vi "SetCurrentSource.vi"() -> ()   [LabVIEW 2024]
uses:
  <vilib>/Instr/_visa.llb/VISA Configure Serial Port (Instr).vi
  <vilib>/Utility/file.llb/Write Delimited Spreadsheet (DBL).vi
panel:
  out "OPT_PWR_MV":dbl format="%#_13g"
  in  "30 dB Power Conversion Factor":dbl=0.0531
  in  "Signal Scaling Factor":dbl
  in  "20 dB Power Conversion Factor":dbl=0.1692
  out "Settings read string":string
  out "Settings reply":string
  out "Settings string":string
  out "ADC read string":string
  in  "Voltage stop (mV)":dbl=3000.0 format="%#_13g"
  out "Saved location and filename":path
  in  "Filename and location":path
  in  "Cal constant":dbl=1.0 format="%#_13g"
  in  "Loop length (ms)":i32=1000
  in  "Voltage step (mV)":dbl=20.0 format="%#_13g"
  out "Voltage (mV)":dbl
  out "Pulse Width":dbl
  out "Frequency":dbl
  out "ACD 2":dbl
  out "ADC 3":dbl
  out "ADC 4":dbl
  out "ADC 1":dbl
  out "RAW 3":dbl
  out "RAW 2":dbl
  out "RAW 4":dbl
  out "RAW 1":dbl
  out "Running?":bool
  in  "ON/OFF":bool
  in  "Voltage start (mV)":dbl=800.0
  in  "Pulse Width (ns)":dbl=3000.0
  in  "Frequency (Hz)":dbl=1000.0
  out "error out":errorcluster
  in  "VISA resource name":refnum<visa-resource-name>
  in  "error in (no error)":errorcluster
  out "VISA resource name out":refnum<visa-resource-name>
  # "mA Readings"
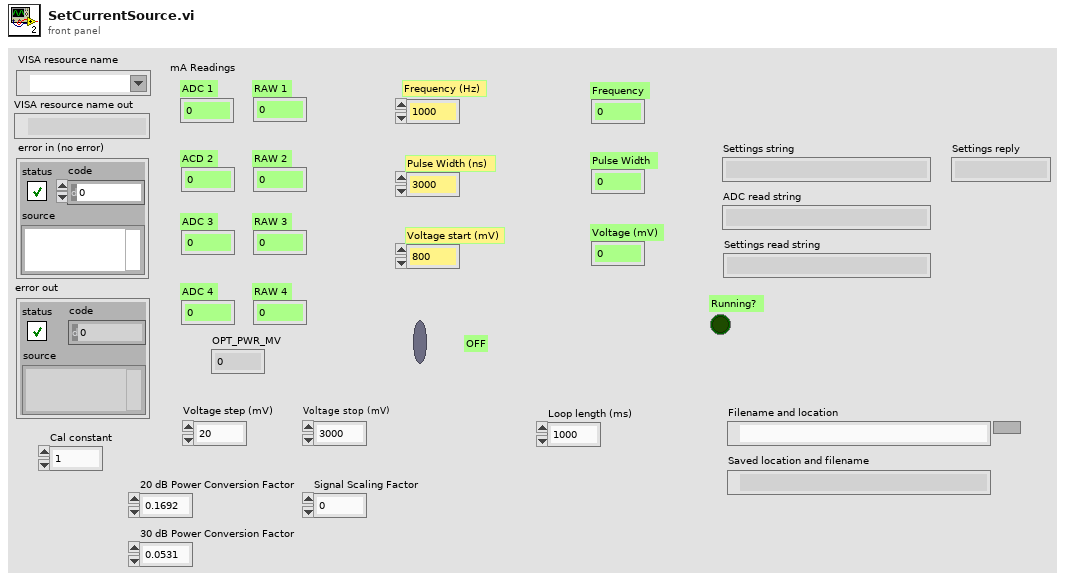
[diagram p1: front panel]
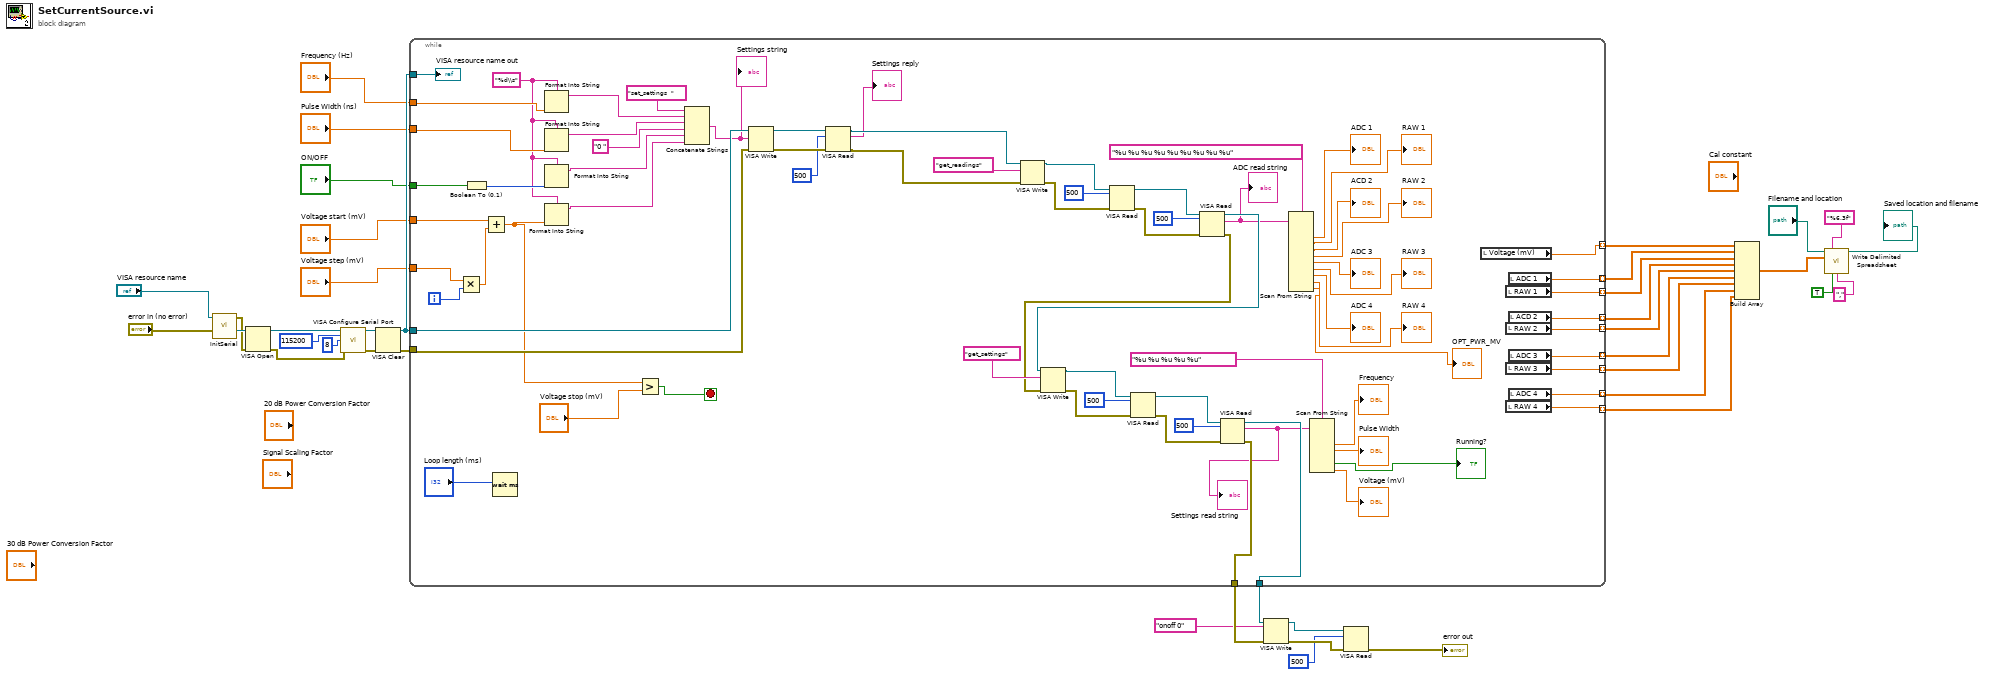
[diagram p0: block diagram]
diagram:
  n1 = call "InitSerial.vi"("error in (no error)"="error in (no error)", "VISA resource name"="VISA resource name") -> ("VISA resource name out"=w37:refnum<visa-resource-name>, "error out"=w29:errorcluster)  [unwired: 8 in]
  n2 = VISA Open(error in (no error)=w29, VISA resource name=w37) -> (VISA resource name=w36:refnum<visa-resource-name>, error out=w28:errorcluster)  [unwired: 3 in]
  n3 = call-poly "VISA Configure Serial Port"("VISA resource name"=w36, "baud rate (9600)"=115200, "data bits (8)"=8, "error in (no error)"=w28) -> ("VISA resource name out"=w32:refnum<visa-resource-name>, "error out"=w33:errorcluster)  [unwired: 10 in]
  n4 = VISA Clear(VISA resource name=w32, error in (no error)=w33) -> (VISA resource name out=w31:refnum<visa-resource-name>, error out=w30:errorcluster)
  n5 = while {
    tunnel: w30 -> [w56]
    tunnel: w31 -> [w112]
    tunnel: w31 -> [w57]
    tunnel: "Voltage start (mV)" -> [w84]
    tunnel: "Pulse Width (ns)" -> [w62]
    tunnel: "Frequency (Hz)" -> [w64]
    tunnel: "Voltage step (mV)" -> [w83]
    tunnel: "ON/OFF" -> [w78]
    tunnel: [w77] -> w22
    tunnel: [w76] -> w21
    tunnel: [w68] -> w10 mode=indexing
    tunnel: [w73] -> w15 mode=indexing
    tunnel: [w65] -> w7 mode=indexing
    tunnel: [w69] -> w11 mode=indexing
    tunnel: [w66] -> w8 mode=indexing
    tunnel: [w70] -> w12 mode=indexing
    tunnel: [w67] -> w9 mode=indexing
    tunnel: [w71] -> w13 mode=indexing
    tunnel: [w72] -> w14 mode=indexing
    i -> [w80]
    stop <- w48 stop-if-true
    w61 = "%d\\s"
    n6 = Multiply(x=w83, y=w80) -> (x*y=w79:dbl)
    n7 = Boolean To (0,1)(Boolean=w78) -> (0, 1=w63:i16)
    n8 = Add(x=w84, y=w79) -> (x+y=w49:dbl)
    n9 = Wait (ms)(milliseconds to wait="Loop length (ms)") -> ()  [unwired: 1 out]
    n10 = Format Into String(format string=w61, w64) -> (resulting string=w59:string)  [unwired: 2 in, 1 out]
    n11 = Format Into String(format string=w61, w62) -> (resulting string=w58:string)  [unwired: 2 in, 1 out]
    n12 = Format Into String(format string=w61, w63) -> (resulting string=w46:string)  [unwired: 2 in, 1 out]
    n13 = Format Into String(format string=w61, w49) -> (resulting string=w47:string)  [unwired: 2 in, 1 out]
    n14 = Greater?(x=w49, y="Voltage stop (mV)") -> (0:w48:bool)
    n15 = Concatenate Strings("set_settings  ", w59, w58, "0 ", w46, w47) -> (w43:string)
    "Settings string" <- w43
    n16 = VISA Write(VISA resource name=w57, write buffer=w43, error in (no error)=w56) -> (VISA resource name out=w54:refnum<visa-resource-name>, error out=w55:errorcluster)  [unwired: 1 out]
    n17 = VISA Read(VISA resource name=w54, byte count=500, error in (no error)=w55) -> (VISA resource name out=w52:refnum<visa-resource-name>, read buffer=→"Settings reply":string, error out=w51:errorcluster)  [unwired: 1 out]
    n18 = VISA Write(VISA resource name=w52, write buffer="get_readings", error in (no error)=w51) -> (VISA resource name out=w107:refnum<visa-resource-name>, error out=w109:errorcluster)  [unwired: 1 out]
    n19 = VISA Read(VISA resource name=w107, byte count=500, error in (no error)=w109) -> (VISA resource name out=w104:refnum<visa-resource-name>, error out=w106:errorcluster)  [unwired: 2 out]
    n20 = VISA Read(VISA resource name=w104, byte count=500, error in (no error)=w106) -> (VISA resource name out=w87:refnum<visa-resource-name>, read buffer=w44:string, error out=w86:errorcluster)  [unwired: 1 out]
    "ADC read string" <- w44
    n21 = VISA Write(VISA resource name=w87, write buffer="get_settings", error in (no error)=w86) -> (VISA resource name out=w95:refnum<visa-resource-name>, error out=w94:errorcluster)  [unwired: 1 out]
    n22 = VISA Read(VISA resource name=w95, byte count=500, error in (no error)=w94) -> (VISA resource name out=w97:refnum<visa-resource-name>, error out=w96:errorcluster)  [unwired: 2 out]
    n23 = VISA Read(VISA resource name=w97, byte count=500, error in (no error)=w96) -> (VISA resource name out=w76:refnum<visa-resource-name>, read buffer=w41:string, error out=w77:errorcluster)  [unwired: 1 out]
    "Settings read string" <- w41
    n24 = Scan From String(format string="%u %u %u %u %u %u %u %u %u", input string=w44) -> (output 1=→"ADC 1":dbl, output 2=→"RAW 1":dbl, output 3=→"ACD 2":dbl, output 4=→"RAW 2":dbl, output 5=→"ADC 3":dbl, output 6=→"RAW 3":dbl, output 7=→"ADC 4":dbl, output 8=→"RAW 4":dbl, output 9=→"OPT_PWR_MV":dbl)  [unwired: 11 in, 3 out]
    n25 = Scan From String(format string="%u %u %u %u %u", input string=w41) -> (output 1=→"Frequency":dbl, output 2=→"Pulse Width":dbl, output 4=→"Running?":bool, output 5=→"Voltage (mV)":dbl)  [unwired: 8 in, 3 out]
    n26 = local read "Voltage (mV)"() -> (w73:dbl)
    n27 = local read "RAW 1"() -> (w69:dbl)
    n28 = local read "RAW 2"() -> (w70:dbl)
    n29 = local read "RAW 3"() -> (w71:dbl)
    n30 = local read "RAW 4"() -> (w72:dbl)
    n31 = local read "ADC 1"() -> (w65:dbl)
    n32 = local read "ACD 2"() -> (w66:dbl)
    n33 = local read "ADC 3"() -> (w67:dbl)
    n34 = local read "ADC 4"() -> (w68:dbl)
    "VISA resource name out" <- w112
  }
  n35 = VISA Write(VISA resource name=w21, write buffer="onoff 0", error in (no error)=w22) -> (VISA resource name out=w19:refnum<visa-resource-name>, error out=w18:errorcluster)  [unwired: 1 out]
  n36 = VISA Read(VISA resource name=w19, byte count=500, error in (no error)=w18) -> (error out=→"error out":errorcluster)  [unwired: 3 out]
  n37 = Build Array(w15, w7, w11, w8, w12, w9, w13, w10, w14) -> (w3:dbl[][])
  n38 = call-poly <vilib>:"Write Delimited Spreadsheet.vi"("file path (dialog if empty)"="Filename and location", "format (%.3f)"="%6.3f", "2D data"=w3, "transpose? (no:F)"=TRUE, "delimiter (\\t)"=",") -> ("new file path (Not A Path if cancelled)"=→"Saved location and filename":path)  [unwired: 9 in, 1 out]
